vi "AFG3352X.update services and attribute data for second channel.vi"(0 "i ref in":refnum<vi>, 1 "direction":T3, 2 "service":T2, 3 "ms timeout (10000)":i32=10000, 4 "value":string, 5 "error in (no error)":errorcluster, 7 "quality":T1=enum."on") -> (14 "i ref out":refnum<vi>, 17 "timed out":bool, 19 "error out":errorcluster)   [LabVIEW 2014, in "AFG3352X.lvlib"]
doc: "Updates the DIM service of a value and updates the attribute data."
uses:
  AFG3352X.lvlib
  CS_Core/CSApplicationBaseClasses/AFGBase/AFGBase.directionType.ctl
  CS_Core/CSApplicationBaseClasses/AFGBase/AFGBase.serviceType.ctl
  CSlibraries/UtilityLib/UtilityLib.valueStatus.ctl
  CSlibraries-extern/DimLVEvent/LVDimInterface/LVDimInterface.lvlib
  CS_Core/CSSystem/CoreLib/CoreLib.lvlib
  CS_Core/CSApplicationBaseClasses/AFGBase/AFGBase.lvlib
  CSlibraries/UtilityLib/UtilityLib.lvlib
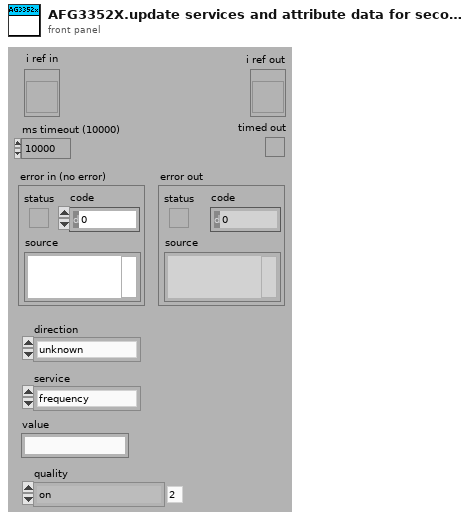
[diagram p1: front panel]
types:
  T1 = typedef "UtilityLib.lvlib/UtilityLib.valueStatus.ctl" = enum16{"no info available", "stand by/off", "on", "warning", "alarm/malfunction", "not implemented", "user action required", "important information", "system default", "control default", "indicator default", "button default"}
  T2 = typedef "AFGBase.lvlib/AFGBase.serviceType.ctl" = enum16{"frequency", "amplitude", "phase", "DCOffset", "enableOutput", "trigger", "waveformType"}
  T3 = typedef "AFGBase.lvlib/AFGBase.directionType.ctl" = enum16{"unknown", "update actual value", "update nominal value", "update both"}
  T4 = typedef "AFG3352X.lvlib/AFG3352X.i attribute.ctl" = cluster{"Act2ndValues":cluster{"frequency":dbl, "amplitude":dbl, "phase":dbl, "DCOffset":dbl, "waveformType":T5, "enableOutput":bool, "trigger":i16[], "serviceIDs":cluster{"frequencyID":i32, "amplitudeID":i32, "phaseID":i32, "DCOffsetID":i32, "waveformTypeID":i32, "enableOutputID":i32, "triggerID":i32}, "waveform":cluster{"data":waveform(dbl), "gain":dbl, "offset":dbl, "repetitionRate":dbl, "sampleRate":dbl}}, "Nom2ndValues":cluster{"frequency":dbl, "amplitude":dbl, "phase":dbl, "DCOffset":dbl, "waveformType":T5, "enableOutput":bool, "trigger":i16[], "serviceIDs":cluster{"frequencyID":i32, "amplitudeID":i32, "phaseID":i32, "DCOffsetID":i32, "waveformTypeID":i32, "enableOutputID":i32, "triggerID":i32}, "waveform":cluster{"data":waveform(dbl), "gain":dbl, "offset":dbl, "repetitionRate":dbl, "sampleRate":dbl}}, "DefaultChannel":i32, "ActAddValues":cluster{"Mode1":u16, "serviceIDs":cluster{"Mode1ID":i32, "Mode2ID":i32, "Burst1ID":i32, "Burst2ID":i32}, "Mode2":u16, "Burst1":i32, "Burst2":i32}, "NomAddValues":cluster{"Mode1":u16, "serviceIDs":cluster{"Mode1ID":i32, "Mode2ID":i32, "Burst1ID":i32, "Burst2ID":i32}, "Mode2 2":u16, "Burst1":i32, "Burst2":i32}, "enableBurstMode":bool}
  T5 = typedef "AFGBase.lvlib/AFGBase.waveformType.ctl" = enum16{"sine", "square", "ramp", "pulse", "noise", "DC", "arbitrary", "triangle", "ramp_up", "ramp_down", "amplitude modulation"}
  T6 = cluster{"frequency":dbl, "amplitude":dbl, "phase":dbl, "DCOffset":dbl, "waveformType":T5, "enableOutput":bool, "trigger":i16[], "serviceIDs":cluster{"frequencyID":i32, "amplitudeID":i32, "phaseID":i32, "DCOffsetID":i32, "waveformTypeID":i32, "enableOutputID":i32, "triggerID":i32}, "waveform":cluster{"data":waveform(dbl), "gain":dbl, "offset":dbl, "repetitionRate":dbl, "sampleRate":dbl}}
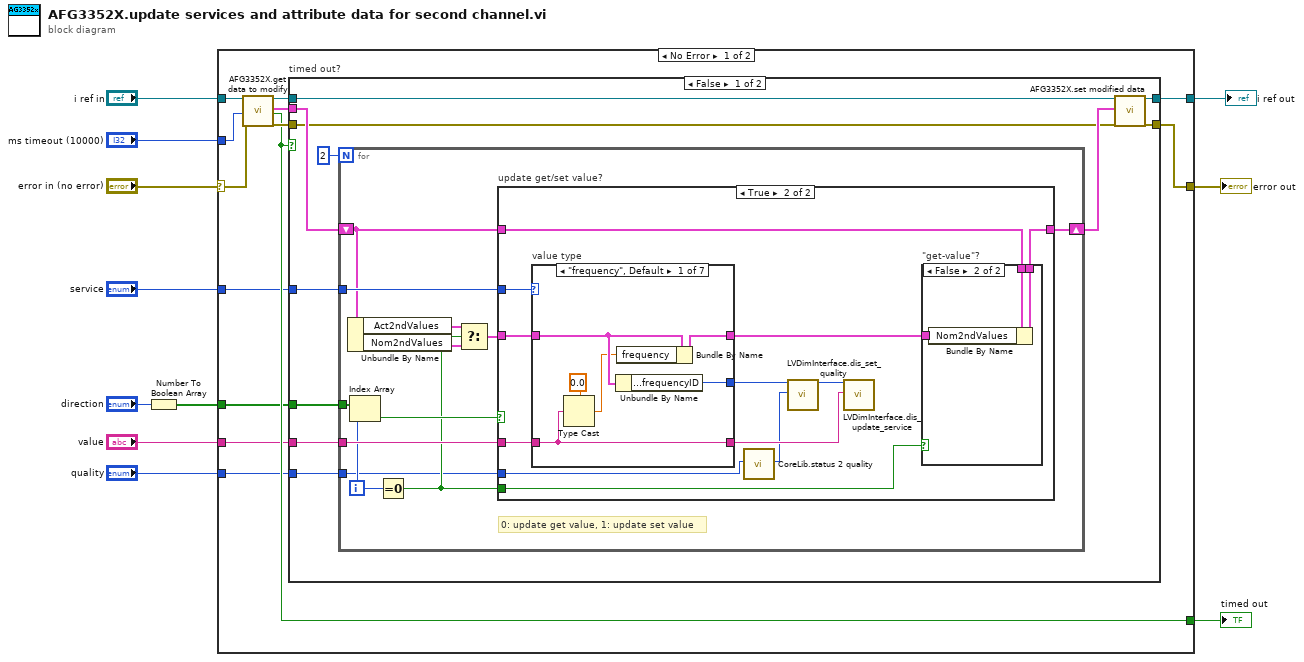
[diagram p0: block diagram]
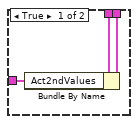
[diagram p3: hidden frame]
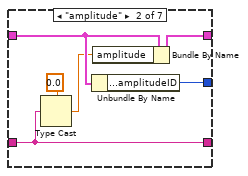
[diagram p4: hidden frame]
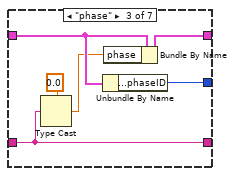
[diagram p5: hidden frame]
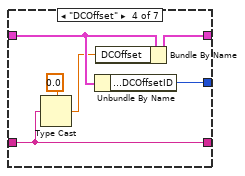
[diagram p6: hidden frame]
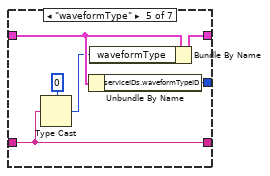
[diagram p7: hidden frame]
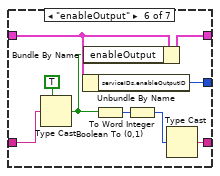
[diagram p8: hidden frame]
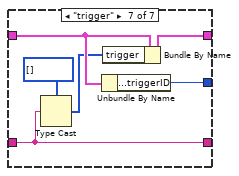
[diagram p9: hidden frame]
diagram:
  n1 = Number To Boolean Array(number="direction") -> (Boolean array=w6:bool[])
  n2 = case shown="No Error" "error in (no error)" {
    selector: "error in (no error)" -> [w22 w115]
    tunnel: [w18 w115] -> w10
    tunnel: "i ref in" -> [w24 w114]
    tunnel: [w20 w114] -> w1
    tunnel: "ms timeout (10000)" -> [w23 _]
    tunnel: [w17 _] -> w8
    tunnel: w6 -> [w15 _]
    tunnel: "service" -> [w14 _]
    tunnel: "value" -> [w13 _]
    tunnel: "quality" -> [w12 _]
    frame No Error {
      n3 = call "AFG3352X.get data to modify.vi"("i ref in"=w24, "ms timeout (10000)"=w23, "error in (no error)"=w22) -> ("i ref out"=w21:refnum<vi>, "i attribute"=w16:T4, "timed out"=w17:bool, "error out"=w19:errorcluster)  [unwired: 13 in]
      n4 = case "timed out?" shown="False" w17 {
        tunnel: w21 -> [w33 w113]
        tunnel: [w35 w113] -> w20
        tunnel: w19 -> [w26 w112]
        tunnel: [w34 w112] -> w18
        tunnel: w16 -> [w30 _]
        tunnel: w15 -> [w31 _]
        tunnel: w14 -> [w29 _]
        tunnel: w13 -> [w28 _]
        tunnel: w12 -> [w25 _]
        frame False {
          n5 = for {
            N: 2 -> [_]
            tunnel: w31 -> [w47]
            tunnel: w29 -> [w45]
            tunnel: w28 -> [w44]
            tunnel: w25 -> [w36]
            shift-right: [w37] -> w27
            shift-left: w30 -> [w39]
            i -> [w43]
            # "0: update get value, 1: update set value"
            n6 = Unbundle By Name(w39) -> ("Act2ndValues"=w42:T6, "Nom2ndValues"=w41:T6)
            n7 = Index Array(array=w47, index=w43) -> (element=w46:bool)
            n8 = Equal To 0?(x=w43) -> (x = 0?=w38:bool)
            n9 = Select(t=w42, s=w38, f=w41) -> (s? t:f=w40:T6)
            n10 = case "update get/set value?" shown="True" w46 {
              tunnel: w45 -> [_ w60]
              tunnel: w44 -> [_ w57]
              tunnel: w40 -> [_ w58]
              tunnel: w39 -> [w48 w56]
              tunnel: w38 -> [_ w54]
              tunnel: [w48 w53] -> w37
              tunnel: w36 -> [_ w52]
              frame False {
              }
              frame True {
                n11 = case "value type" shown="\"frequency\", Default" w60 {
                  tunnel: w58 -> [w71 w77 w83 w89 w95 w104 w110]
                  tunnel: [w72 w78 w84 w90 w96 w105 w111] -> w50
                  tunnel: [w67 w73 w79 w85 w91 w98 w107] -> w59
                  tunnel: w57 -> [w67 w73 w79 w85 w91 w102 w107]
                  tunnel: [w70 w76 w82 w88 w94 w103 w109] -> w55
                  frame "frequency", Default {
                    n12 = Type Cast(type=0.0, x=w67) -> (*(type *) &x=w68:dbl)
                    n13 = Unbundle By Name(w71) -> ("serviceIDs.frequencyID"=w72:i32)
                    n14 = Bundle By Name(cluster=w71, "frequency"=w68) -> (w70:T6)
                  }
                  frame "amplitude" {
                    n15 = Type Cast(type=0.0, x=w73) -> (*(type *) &x=w74:dbl)
                    n16 = Unbundle By Name(w77) -> ("serviceIDs.amplitudeID"=w78:i32)
                    n17 = Bundle By Name(cluster=w77, "amplitude"=w74) -> (w76:T6)
                  }
                  frame "phase" {
                    n18 = Type Cast(type=0.0, x=w79) -> (*(type *) &x=w80:dbl)
                    n19 = Unbundle By Name(w83) -> ("serviceIDs.phaseID"=w84:i32)
                    n20 = Bundle By Name(cluster=w83, "phase"=w80) -> (w82:T6)
                  }
                  frame "DCOffset" {
                    n21 = Type Cast(type=0.0, x=w85) -> (*(type *) &x=w86:dbl)
                    n22 = Unbundle By Name(w89) -> ("serviceIDs.DCOffsetID"=w90:i32)
                    n23 = Bundle By Name(cluster=w89, "DCOffset"=w86) -> (w88:T6)
                  }
                  frame "waveformType" {
                    n24 = Type Cast(type=0, x=w91) -> (*(type *) &x=w92:i32)
                    n25 = Unbundle By Name(w95) -> ("serviceIDs.waveformTypeID"=w96:i32)
                    n26 = Bundle By Name(cluster=w95, "waveformType"=w92) -> (w94:T6)
                  }
                  frame "enableOutput" {
                    n27 = Type Cast(type=TRUE, x=w102) -> (*(type *) &x=w100:bool)
                    n28 = Unbundle By Name(w104) -> ("serviceIDs.enableOutputID"=w105:i32)
                    n29 = Bundle By Name(cluster=w104, "enableOutput"=w100) -> (w103:T6)
                    n30 = Boolean To (0,1)(Boolean=w100) -> (0, 1=w99:i16)
                    n31 = To Word Integer(number=w99) -> (16bit integer=w97:i16)
                    n32 = Type Cast(x=w97) -> (*(type *) &x=w98:string)  [unwired: 1 in]
                  }
                  frame "trigger" {
                    n33 = Type Cast(type=i16[] [], x=w107) -> (*(type *) &x=w108:i16[])
                    n34 = Unbundle By Name(w110) -> ("serviceIDs.triggerID"=w111:i32)
                    n35 = Bundle By Name(cluster=w110, "trigger"=w108) -> (w109:T6)
                  }
                }
                n36 = call "CoreLib.status 2 quality.vi"("valueStatus"=w52) -> ("quality"=w51:i32)  [unwired: 18 in]
                n37 = call "LVDimInterface.dis_set_quality.vi"("my_serviceID"=w50, "quality"=w51) -> ("my_serviceID (out)"=w49:i32)  [unwired: 16 in, 1 out]
                n38 = call "LVDimInterface.dis_update_service.vi"("my_serviceID"=w49, "data"=w59) -> ()  [unwired: 15 in, 3 out]
                n39 = case "\"get-value\"?" shown="False" w54 {
                  tunnel: w56 -> [w63 w66]
                  tunnel: w55 -> [w62 w65]
                  tunnel: [w61 w64] -> w53
                  frame True {
                    n40 = Bundle By Name(cluster=w63, "Act2ndValues"=w62) -> (w61:T4)
                  }
                  frame False {
                    n41 = Bundle By Name(cluster=w66, "Nom2ndValues"=w65) -> (w64:T4)
                  }
                }
              }
            }
          }
          n42 = call "AFG3352X.set modified data.vi"("i ref in"=w33, "i attribute"=w27, "error in (no error)"=w26) -> ("i ref out"=w35:refnum<vi>, "error out"=w34:errorcluster)  [unwired: 15 in]
        }
        frame True {
        }
      }
    }
    frame Error {
    }
  }
  "error out" <- w10
  "timed out" <- w8
  "i ref out" <- w1
